vi "GP275 Convectron Guage.vi"() -> ()   [LabVIEW 2011]
panel:
  in  "Input Byte 4":u8
  in  "Input Byte 3":u8
  in  "Stop Button":bool
  out "Pressure (Torr)":sgl
  out "Warning":bool
  out "Alarm":bool
  in  "Input Byte 2":u8
  in  "Input Byte 1":u8
  in  "Input Byte 0":u8
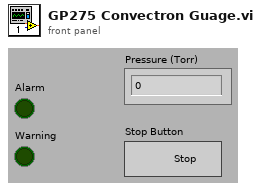
[diagram p1: front panel]
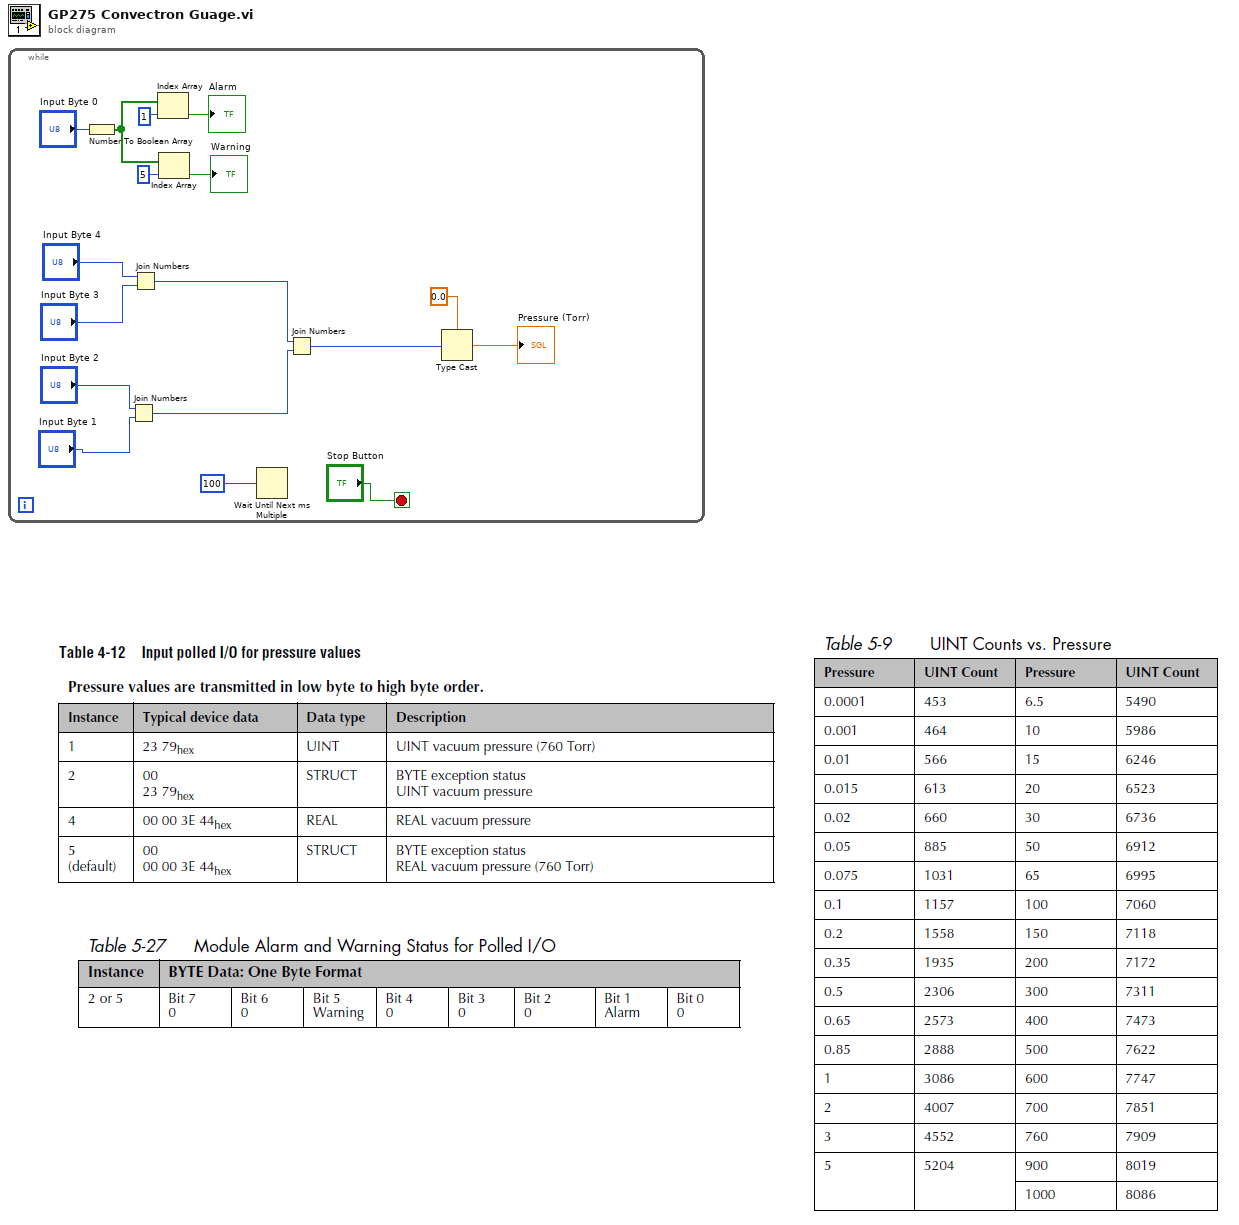
[diagram p0: block diagram]
diagram:
  n1 = while {
    stop <- "Stop Button" stop-if-true
    n2 = Number To Boolean Array(number="Input Byte 0") -> (Boolean array=w14:bool[])
    n3 = Join Numbers(hi="Input Byte 2", lo="Input Byte 1") -> ((hi.lo)=w7:u16)
    n4 = Join Numbers(hi="Input Byte 4", lo="Input Byte 3") -> ((hi.lo)=w6:u16)
    n5 = Index Array(array=w14, index=1) -> (element=→"Alarm":bool)
    n6 = Index Array(array=w14, index=5) -> (element=→"Warning":bool)
    n7 = Wait Until Next ms Multiple(millisecond multiple=u32 100) -> ()  [unwired: 1 out]
    n8 = Join Numbers(hi=w6, lo=w7) -> ((hi.lo)=w5:u32)
    n9 = Type Cast(type=sgl 0.0, x=w5) -> (*(type *) &x=→"Pressure (Torr)":sgl)
  }
